vi "FTW-Ether-CreateSubscriber.vi"(5 "Publisher Address":string, 7 "Publisher Identity":string, 11 "error in":errorcluster) -> (4 "Subscriber Endpoint":refnum<class "FTW-Endpoint.lvclass">, 10 "Incoming Requests":refnum<event-registration>, 15 "error out":errorcluster)   [LabVIEW 2013, in "FTW-Actor.lvlib" / "FTW-Ether.lvclass"]
uses:
  FTW-Ether.lvclass
  Endpoint/FTW-Endpoint.lvclass
  Message/Request/FTW-Message-IncomingRequest.lvclass
  FTW-Ether-EndpointType.ctl
panel:
  # "Inputs"
  # "Outputs"
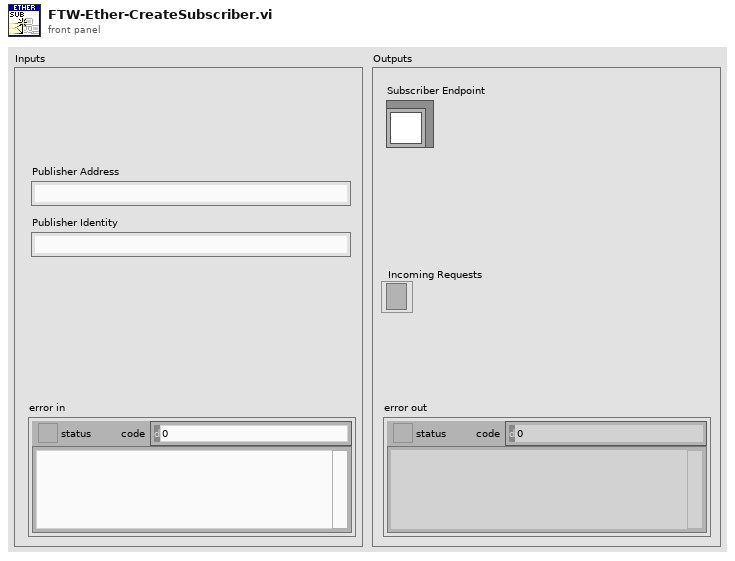
[diagram p1: front panel]
types:
  T1 = typedef "FTW-Actor.lvlib/FTW-Ether.lvclass/FTW-Ether-EndpointType.ctl" = enum16{"Server", "Client", "Publisher", "Subscriber"}
  T2 = typedef "FTW-Actor.lvlib/FTW-Ether.lvclass/FTW-Ether-MessageTransportScheme.ctl" = enum16{"LabVIEW Queues (lvq://)", "LabVIEW Notifiers (lvn://)", "LabVIEW Network Streams (lvns://)"}
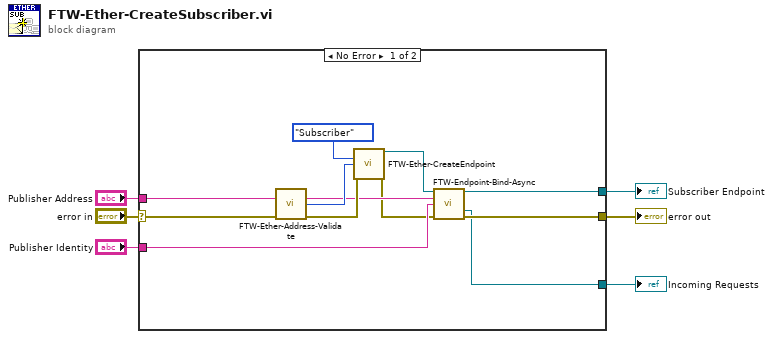
[diagram p0: block diagram]
diagram:
  n1 = case shown="No Error" "error in" {
    selector: "error in" -> [w15 w19]
    tunnel: [w18 _] -> w2
    tunnel: [w17 w19] -> w3
    tunnel: "Publisher Address" -> [w14 _]
    tunnel: "Publisher Identity" -> [w11 _]
    tunnel: [w10 _] -> w1
    frame No Error {
      n2 = call "FTW-Ether-Address-Validate.vi"("Address"=w14, "error in"=w15) -> ("Sanitized Address"=w12:string, "Message Transport Scheme"=w13:T2, "error out"=w16:errorcluster)  [unwired: 11 in]
      n3 = call "FTW-Ether-CreateEndpoint.vi"("Endpoint Type"=FTW-Ether-EndpointType."Subscriber", "Message Transport Scheme"=w13, "error in"=w16) -> ("FTW Endpoint"=w9:refnum<class "FTW-Endpoint.lvclass">, "error out"=w7:errorcluster)  [unwired: 11 in]
      n4 = call-dynamic "FTW-Endpoint-Bind-Async.vi"("FTW Endpoint"=w9, "Endpoint Address"=w12, "Requested Identity"=w11, "error in"=w7) -> ("FTW Endpoint out"=w18:refnum<class "FTW-Endpoint.lvclass">, "Incoming Requests"=w10:refnum<event-registration>, "error out"=w17:errorcluster)  [unwired: 7 in, 2 out]
    }
    frame Error {
    }
  }
  "error out" <- w3
  "Subscriber Endpoint" <- w2
  "Incoming Requests" <- w1
